vi "Start IP Reporter.vi"(4 "ignore Gateway IP?(T)":bool=TRUE, 6 "Load From File(F)":bool, 8 "error in (no error)":errorcluster, 10 "Information":string, 11 "Setttings":T1={"address"="234.5.6.7", "receiver port"=58432, "Ignore Gateway IP"=TRUE, "HostName"=""}) -> (0 "error out":errorcluster)   [LabVIEW 2017]
uses:
  _Typedef/Def-IniSettings -- Cluster.ctl
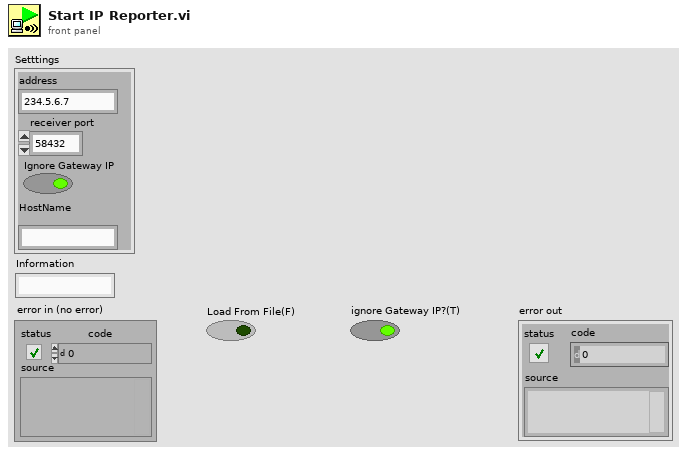
[diagram p1: front panel]
types:
  T1 = typedef "Def-IniSettings -- Cluster.ctl" = cluster{"address":string, "receiver port":u16, "Ignore Gateway IP":bool, "HostName":string}
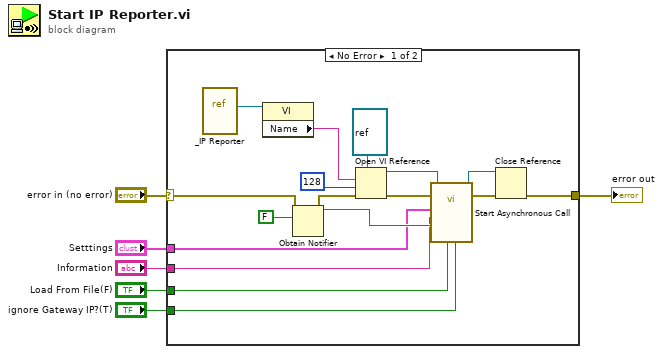
[diagram p0: block diagram]
diagram:
  n1 = case shown="No Error" "error in (no error)" {
    selector: "error in (no error)" -> [w23 w24]
    tunnel: [w16 w24] -> w5
    tunnel: "Setttings" -> [w10 _]
    tunnel: "Load From File(F)" -> [w9 _]
    tunnel: "ignore Gateway IP?(T)" -> [w8 _]
    tunnel: "Information" -> [w7 _]
    frame No Error {
      n2 = vi-ref "_IP Reporter.vi"() -> (w21:refnum<vi>)
      n3 = property class="VI"(reference=w21) -> ("Name"=w20:string)  [unwired: 1 in, 2 out]
      n4 = Obtain Notifier(notification data type=FALSE, error in (no error)=w23) -> (notifier out=w11:refnum<notifier>, error out=w13:errorcluster)  [unwired: 2 in, 1 out]
      n5 = Open VI Reference(type specifier VI Refnum (for type only)=refnum<vi> refnum, vi path=w20, options=128, error in (no error)=w13) -> (vi reference=w14:refnum<vi>, error out=w22:errorcluster)  [unwired: 2 in]
      n6 = call-by-ref "Start Asynchronous Call"(reference=w14, error in=w22, "ignore Gateway IP?(T)"=w8, "Load From File(F)"=w9, "WatchDog(notifier)"=w11, "Information"=w7, "Setttings"=w10) -> (reference out=w15:refnum<vi>, error out=w18:errorcluster)  [unwired: 6 in, 1 out]
      n7 = Close Reference(reference=w15, error in (no error)=w18) -> (error out=w16:errorcluster)
    }
    frame Error {
    }
  }
  "error out" <- w5
